vi "Query Wavelength Calibration Coefficient.vi"(8 "error in (no error)":errorcluster, 11 "VISA resource name":refnum<visa-resource-name>) -> (0 "error out":errorcluster, 1 "2nd Order Wavelength Calibration Coefficient":dbl format="%#_15g", 2 "1st Order Wavelength Calibration Coefficient":dbl format="%#_15g", 3 "VISA resource name out":refnum<visa-resource-name>, 4 "3rd Order Wavelength Calibration Coefficient":dbl format="%#_15g", 5 "0th Order Wavelength Calibration Coefficient":dbl format="%#_15g")   [LabVIEW 2012, in "Ocean Optics 2000 4000.lvlib"]
doc: "Returns the wavelength calibration coefficients stored in the EEPROM. These coefficients are used to calibrate the wavelength based on the pixel number."
uses:
  Ocean Optics 2000 4000.lvlib
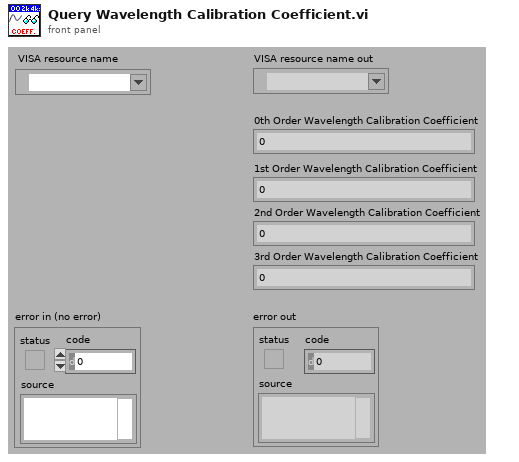
[diagram p1: front panel]
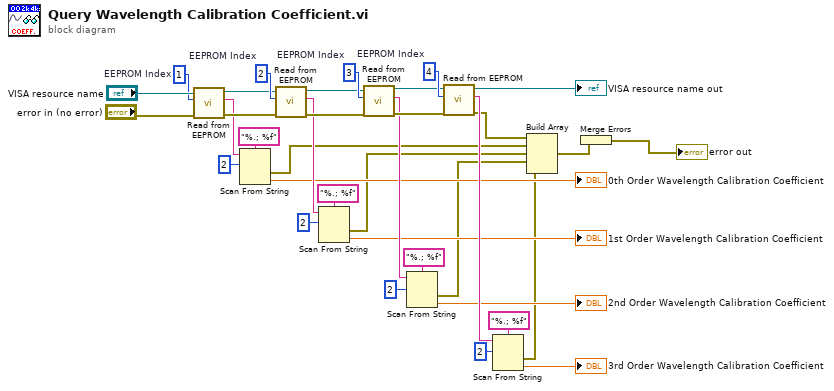
[diagram p0: block diagram]
diagram:
  w31 = u8 4  # EEPROM Index
  w32 = u8 3  # EEPROM Index
  w33 = u8 2  # EEPROM Index
  w34 = u8 1  # EEPROM Index
  n1 = call "Read from EEPROM.vi"("error in (no error)"="error in (no error)", "EEPROM Index"=w34, "VISA resource name"="VISA resource name") -> ("error out"=w29:errorcluster, "ASCII Data"=w2:string, "VISA resource name out"=w30:refnum<visa-resource-name>)  [unwired: 6 out]
  n2 = Scan From String(format string="%.; %f", input string=w2, initial scan location=u32 2) -> (error out=w6:errorcluster, output 1=→"0th Order Wavelength Calibration Coefficient":dbl)  [unwired: 1 in, 3 out]
  n3 = call "Read from EEPROM.vi"("error in (no error)"=w29, "EEPROM Index"=w33, "VISA resource name"=w30) -> ("error out"=w27:errorcluster, "ASCII Data"=w23:string, "VISA resource name out"=w28:refnum<visa-resource-name>)  [unwired: 6 out]
  n4 = Scan From String(format string="%.; %f", input string=w23, initial scan location=u32 2) -> (error out=w5:errorcluster, output 1=→"1st Order Wavelength Calibration Coefficient":dbl)  [unwired: 1 in, 3 out]
  n5 = call "Read from EEPROM.vi"("error in (no error)"=w27, "EEPROM Index"=w32, "VISA resource name"=w28) -> ("error out"=w25:errorcluster, "ASCII Data"=w20:string, "VISA resource name out"=w26:refnum<visa-resource-name>)  [unwired: 6 out]
  n6 = Scan From String(format string="%.; %f", input string=w20, initial scan location=u32 2) -> (error out=w4:errorcluster, output 1=→"2nd Order Wavelength Calibration Coefficient":dbl)  [unwired: 1 in, 3 out]
  n7 = call "Read from EEPROM.vi"("error in (no error)"=w25, "EEPROM Index"=w31, "VISA resource name"=w26) -> ("error out"=w8:errorcluster, "ASCII Data"=w17:string, "VISA resource name out"=→"VISA resource name out":refnum<visa-resource-name>)  [unwired: 6 out]
  n8 = Scan From String(format string="%.; %f", input string=w17, initial scan location=u32 2) -> (error out=w3:errorcluster, output 1=→"3rd Order Wavelength Calibration Coefficient":dbl)  [unwired: 1 in, 3 out]
  n9 = Build Array(w8, w6, w5, w4, w3) -> (w1:errorcluster[])
  n10 = Merge Errors(w1) -> (→"error out":errorcluster)
